vi "connect to db.vi"(8 "error in (no error)":errorcluster, 11 "database in":refnum<class "database.lvclass">) -> (0 "error out":errorcluster, 3 "database out":refnum<class "database.lvclass">)   [LabVIEW 2018, in "database.lvclass"]
uses:
  database.lvclass
  database.lvclass/database.ctl
  <vilib>/addons/database/Connection.llb/DB Tools Open Connec (String).vi
  <vilib>/addons/database/NI_Database_API.lvlib
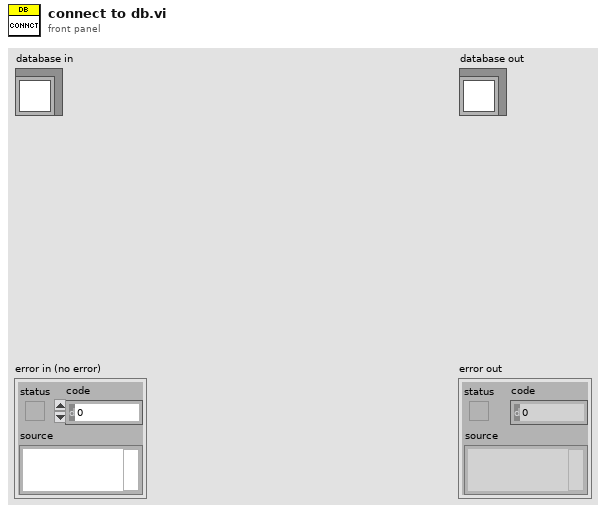
[diagram p1: front panel]
types:
  T1 = typedef "NI_Database_API.lvlib/Conn ObjectReference.ctl" = refnum<k1>
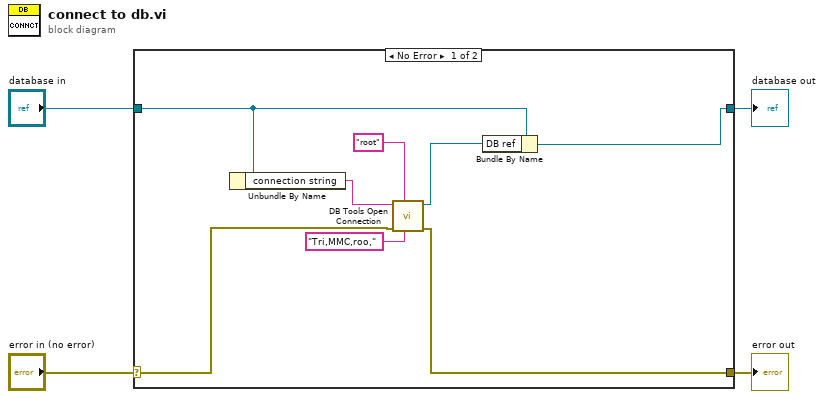
[diagram p0: block diagram]
diagram:
  n1 = case shown="No Error" "error in (no error)" {
    selector: "error in (no error)" -> [w9 w14]
    tunnel: [w8 w14] -> w3
    tunnel: [w6 w13] -> w1
    tunnel: "database in" -> [w7 w13]
    frame No Error {
      n2 = Unbundle By Name(w7) -> ("connection string"=w12:string)
      n3 = call-poly <vilib>:"DB Tools Open Connection.vi"("password"="Tri,MMC,roo,", "userID"="root", "error in (no error)"=w9, "connection information"=w12) -> ("error out"=w8:errorcluster, "connection reference"=w5:T1)  [unwired: 4 in]
      n4 = Bundle By Name(cluster=w7, "DB ref"=w5) -> (w6:refnum<class "database.lvclass">)
    }
    frame Error {
    }
  }
  "error out" <- w3
  "database out" <- w1
